vi "String_Field.vi"(11 "String":string="Set Magnetic Field 0.500Tesla at 0.050Tesla/min, Linear, Persistent, Wait") -> (0 "F.Mode":i32(ring) items=["Persistent", "Driven"], 1 "F.Approach":i32(ring) items=["Linear", "NoOvershoot", "Oscillate"], 2 "Rate":dbl, 3 "Field":dbl, 4 "H.Wait Stability":bool)   [LabVIEW 2017]
panel:
  out "subString":string
  # "Set Magnetic Field 1000.000Tesla at 100.000Tesla/min, Linear, Persistent, Wait"
  # "Set Magnetic Field 0.500Tesla at 0.005Tesla/min, Linear, Persistent, NOWait"
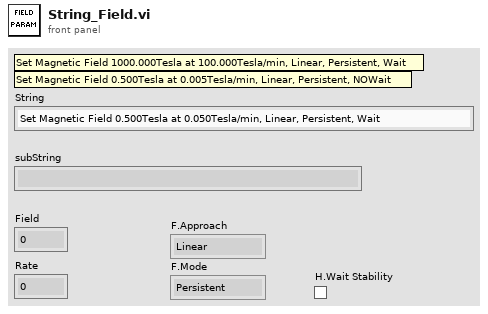
[diagram p1: front panel]
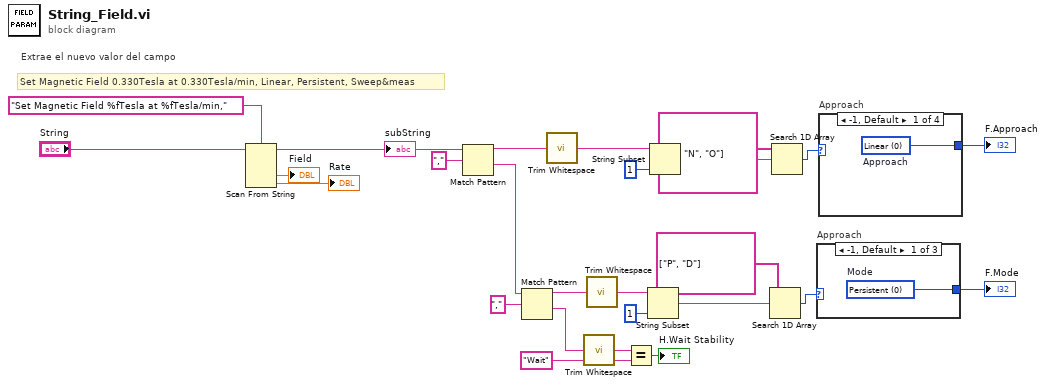
[diagram p0: block diagram]
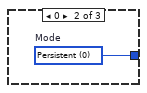
[diagram p2: hidden frame]
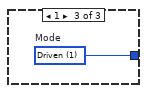
[diagram p3: hidden frame]
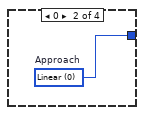
[diagram p4: hidden frame]
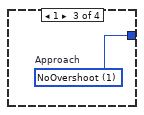
[diagram p5: hidden frame]
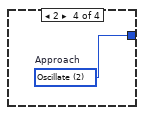
[diagram p6: hidden frame]
diagram:
  # "Set Magnetic Field 0.330Tesla at 0.330Tesla/min, Linear, Persistent, Sweep&meas"
  # "Extrae el nuevo valor del campo"
  n1 = Scan From String(format string="Set Magnetic Field %fTesla at %fTesla/min,", input string="String") -> (remaining string=w1:string, output 1=→"Field":dbl, output 2=→"Rate":dbl)  [unwired: 4 in, 2 out]
  "subString" <- w1
  n2 = Match Pattern(string=w1, regular expression=",") -> (before substring=w7:string, after substring=w11:string)  [unwired: 1 in, 2 out]
  n3 = Match Pattern(string=w11, regular expression=",") -> (before substring=w5:string, after substring=w3:string)  [unwired: 1 in, 2 out]
  n4 = call <vilib>:"Trim Whitespace.vi"("string"=w7) -> ("trimmed string"=w6:string)  [unwired: 1 in]
  n5 = call <vilib>:"Trim Whitespace.vi"("string"=w3) -> ("trimmed string"=w2:string)  [unwired: 1 in]
  n6 = call <vilib>:"Trim Whitespace.vi"("string"=w5) -> ("trimmed string"=w4:string)  [unwired: 1 in]
  n7 = Equal?(x=w2, y="Wait" ("after substring")) -> (x = y?=→"H.Wait Stability":bool)
  n8 = String Subset(string=w4, length (rest)=1 ("length (rest)")) -> (substring=w18:string)  [unwired: 1 in]
  n9 = String Subset(string=w6, length (rest)=1 ("length (rest)")) -> (substring=w21:string)  [unwired: 1 in]
  n10 = Search 1D Array(1D array=string[] ["P", "D"], element=w18) -> (index of element=w19:i32)  [unwired: 1 in]
  n11 = Search 1D Array(1D array=string[] ["L", "N", "O"], element=w21) -> (index of element=w20:i32)  [unwired: 1 in]
  n12 = case "Approach" shown="-1, Default" w19 {
    tunnel: [w27 w28 w29] -> w15
    frame -1, Default {
      w27 = 0 items=["Persistent", "Driven"]  # Mode
    }
    frame 0 {
      w28 = 0 items=["Persistent", "Driven"]  # Mode
    }
    frame 1 {
      w29 = 1 items=["Persistent", "Driven"]  # Mode
    }
  }
  "F.Mode" <- w15
  n13 = case "Approach" shown="-1, Default" w20 {
    tunnel: [w30 w31 w32 w33] -> w14
    frame -1, Default {
      w30 = 0 items=["Linear", "NoOvershoot", "Oscillate"]  # Approach
    }
    frame 0 {
      w31 = 0 items=["Linear", "NoOvershoot", "Oscillate"]  # Approach
    }
    frame 1 {
      w32 = 1 items=["Linear", "NoOvershoot", "Oscillate"]  # Approach
    }
    frame 2 {
      w33 = 2 items=["Linear", "NoOvershoot", "Oscillate"]  # Approach
    }
  }
  "F.Approach" <- w14
